vi "The ChapR.vi"(9 "Position":u8=49, 10 "Alliance":u8=66, 11 "TeamNo":u16=2468) -> ()   [LabVIEW 2013]
uses:
  ChapR Packet.ctl
  <vilib>/Instr/_visa.llb/VISA Configure Serial Port (Instr).vi
panel:
  out "error out 3":errorcluster
  in  "connection ID":refnum<k16>
  out "error out 2":errorcluster
  out "# elements 2":u32
  out "# elements":u32
  out "error out":errorcluster
  out "value 2":T1
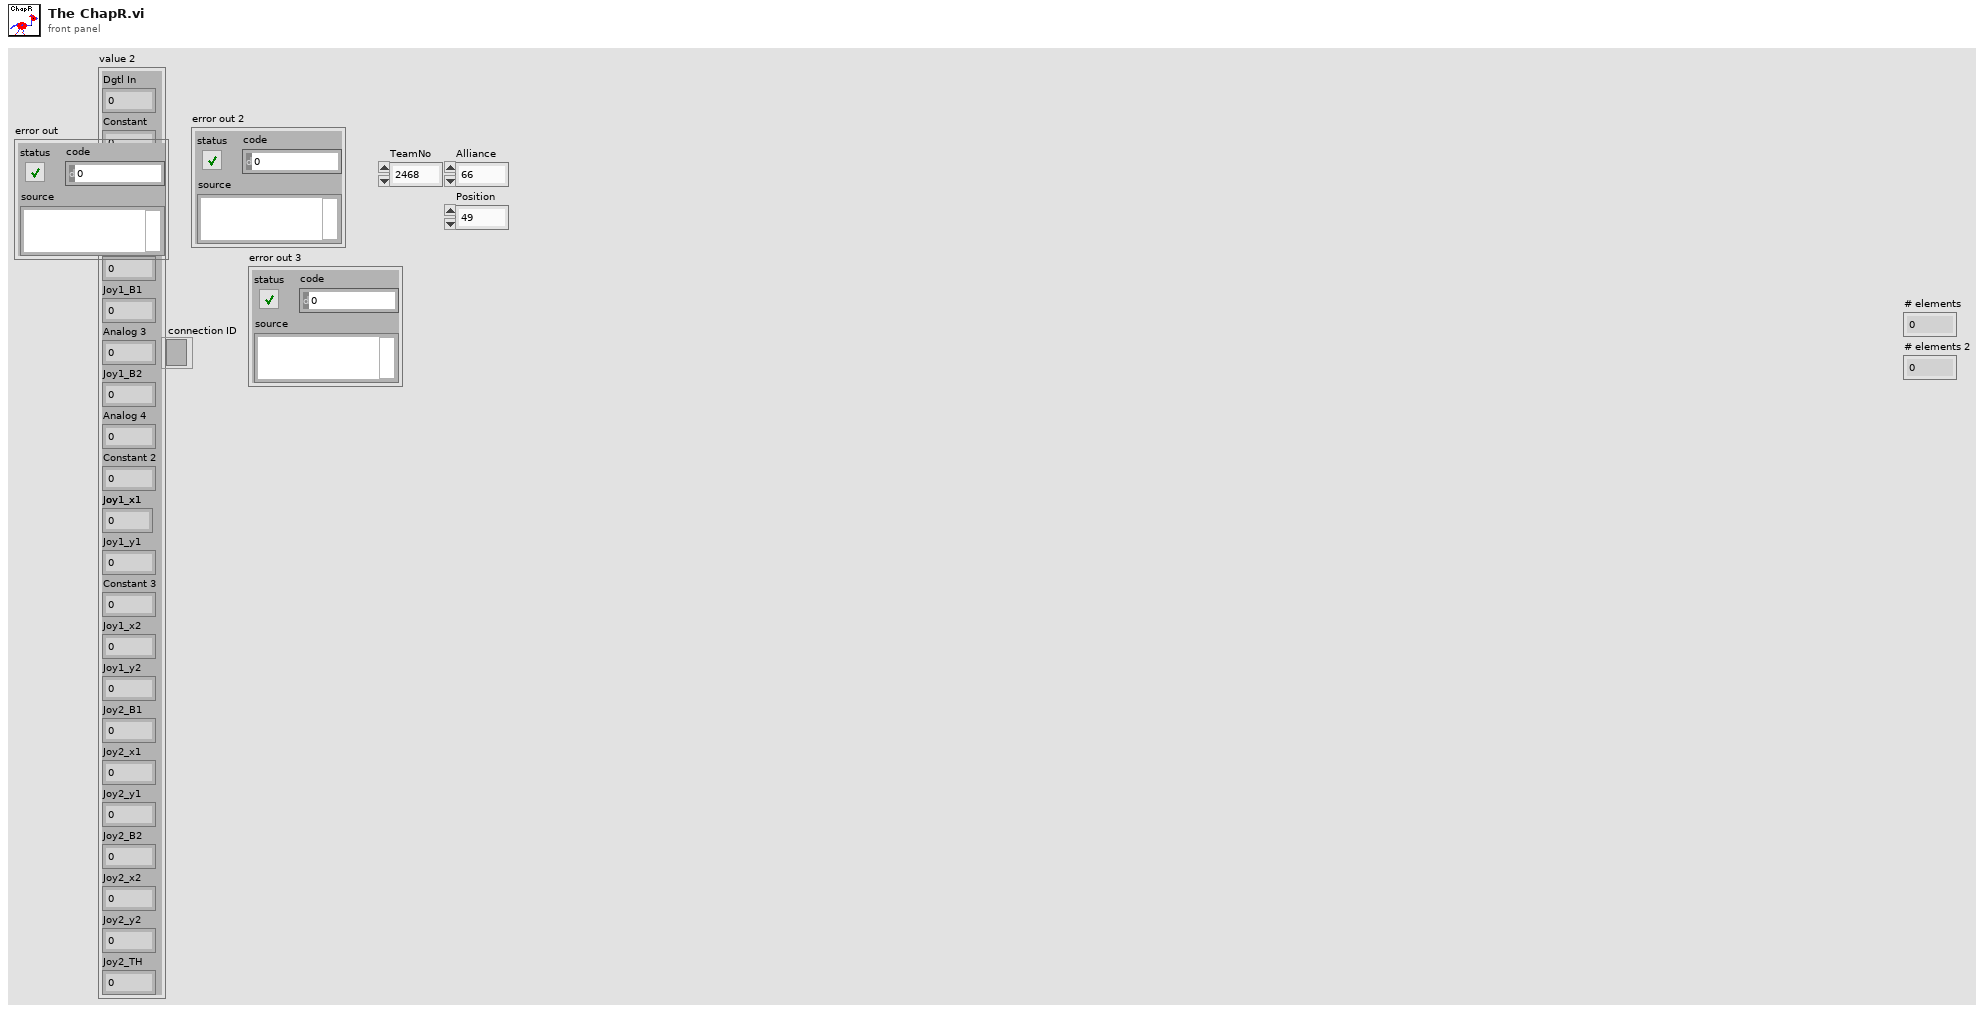
[diagram p1: front panel]
types:
  T1 = typedef "ChapR Packet.ctl" = cluster{"Dgtl In":u8, "Constant":u8, "Analog 1":u16, "Joy1_TH":u8, "Analog 2":u16, "Joy1_B1":u8, "Analog 3":u16, "Joy1_B2":u8, "Analog 4":u16, "Constant 2":u8, "Joy1_x1":i8, "Joy1_y1":i8, "Constant 3":u8, "Joy1_x2":i8, "Joy1_y2":i8, "Joy2_B1":u8, "Joy2_x1":i8, "Joy2_y1":i8, "Joy2_B2":u8, "Joy2_x2":i8, "Joy2_y2":i8, "Joy2_TH":u8}
  T2 = cluster{"read mode":enum16{"polling", "blocking"}, "write mode":enum16{"polling", "blocking"}}
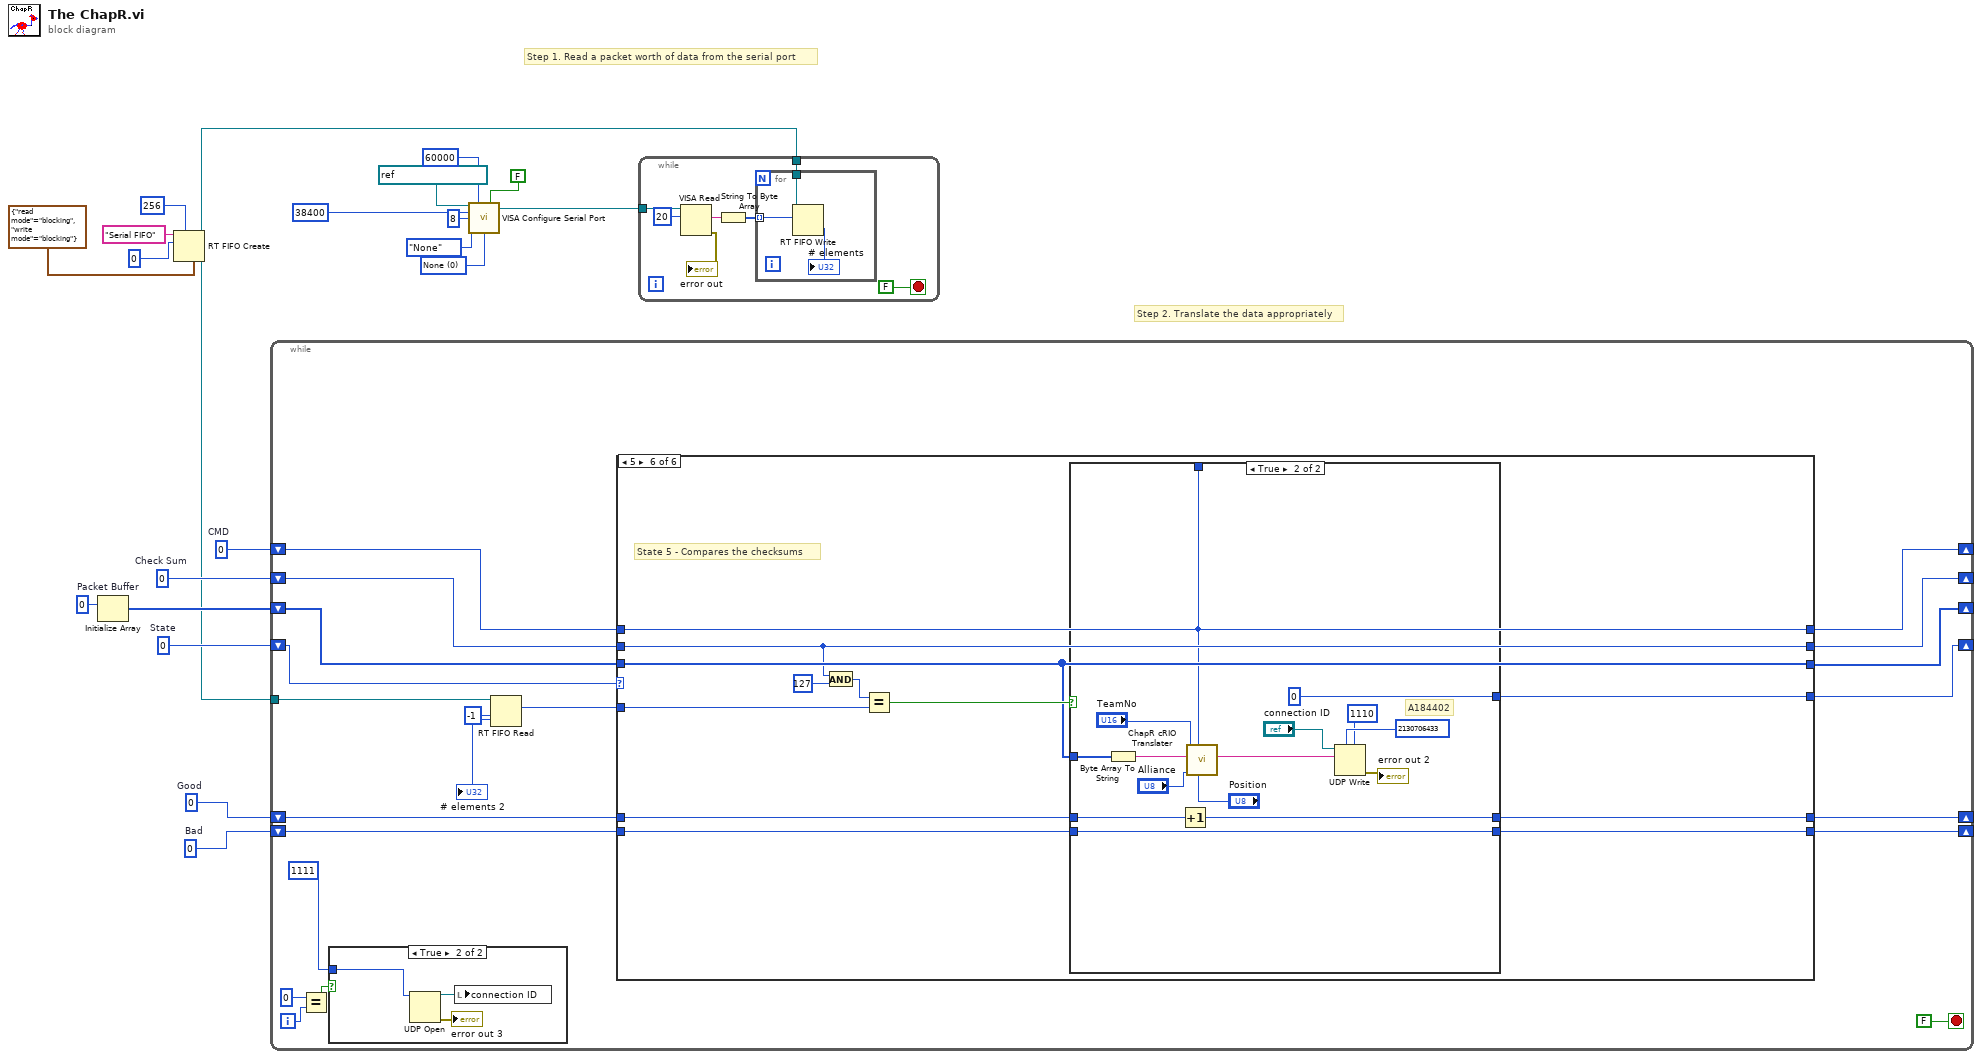
[diagram p0: block diagram]
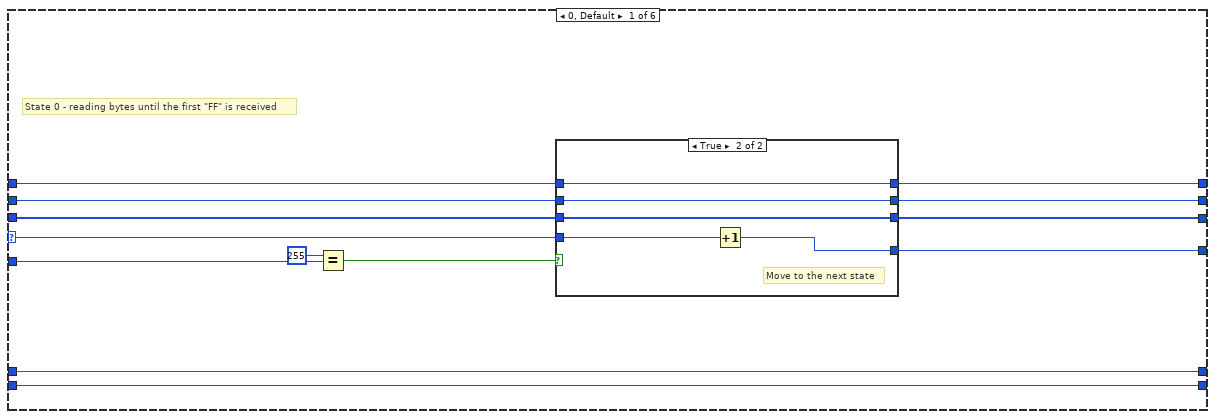
[diagram p3: hidden frame]
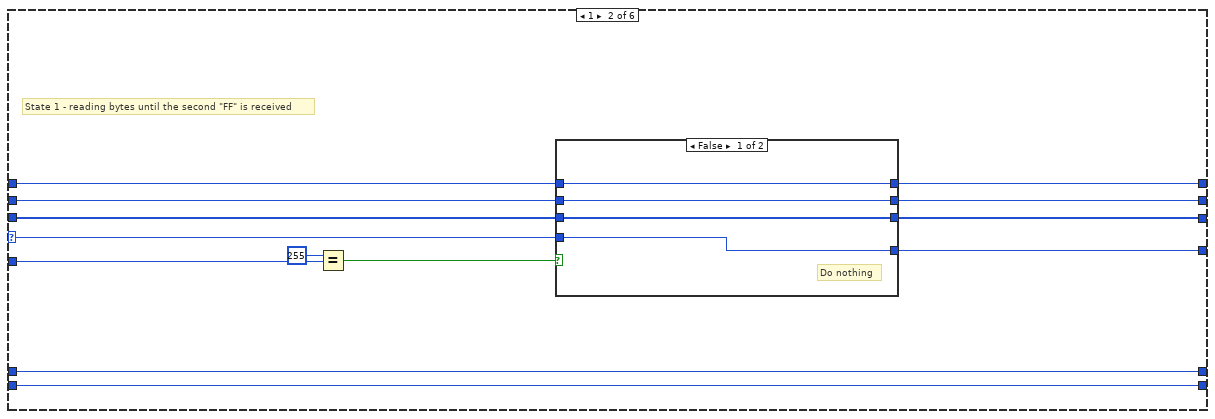
[diagram p5: hidden frame]
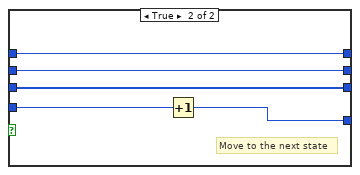
[diagram p6: hidden frame]
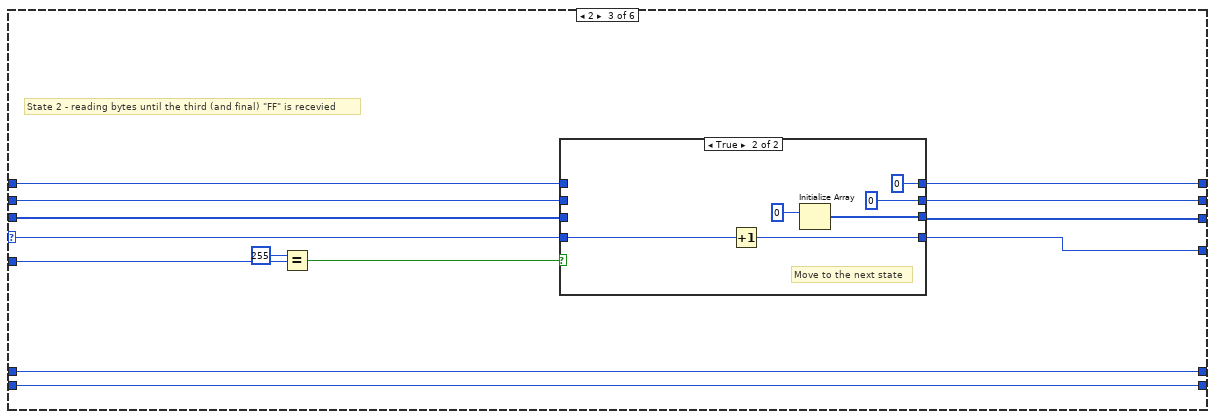
[diagram p7: hidden frame]
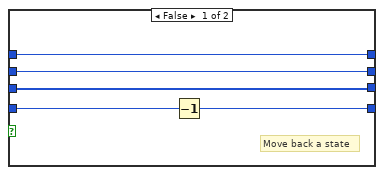
[diagram p8: hidden frame]
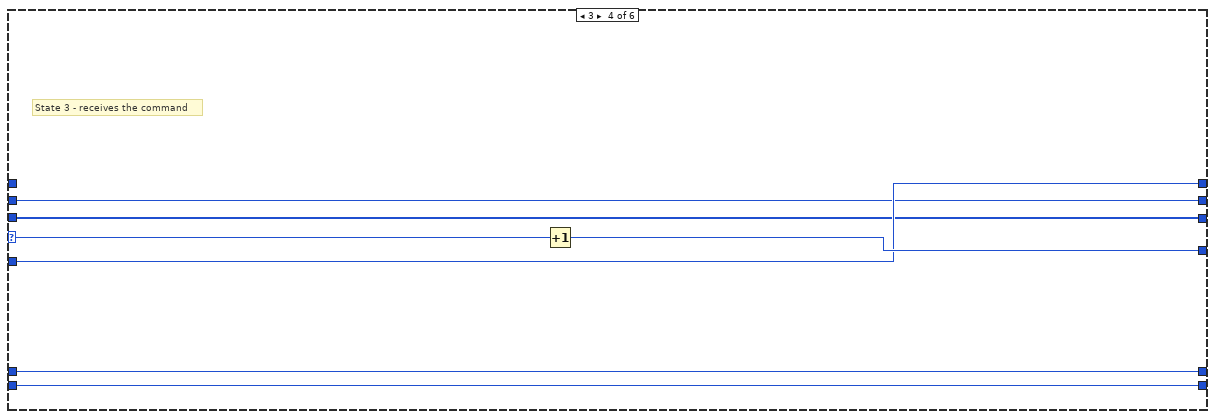
[diagram p9: hidden frame]
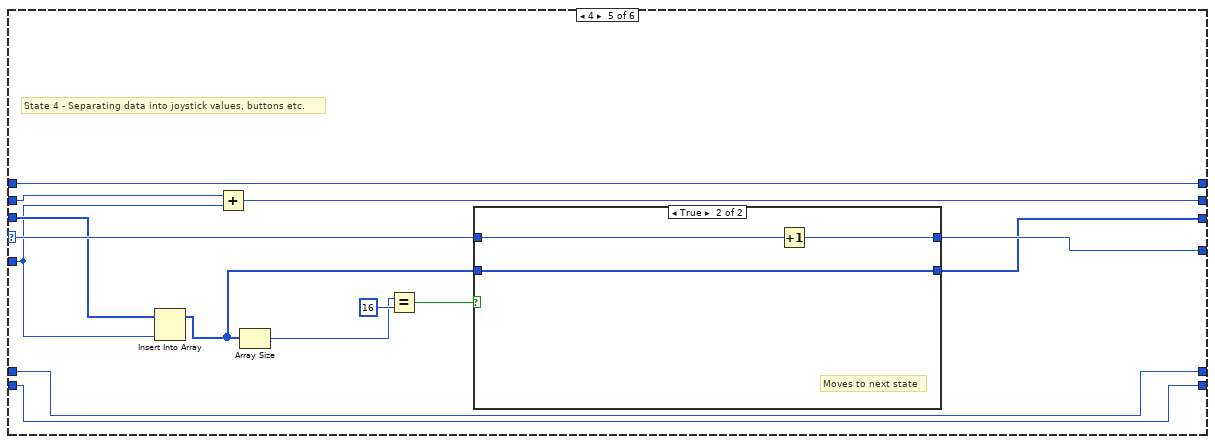
[diagram p10: hidden frame]
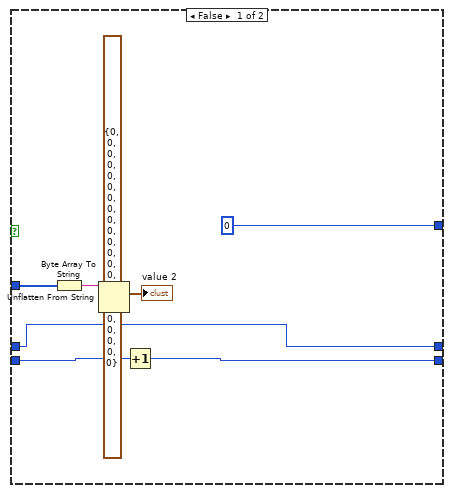
[diagram p12: hidden frame]
diagram:
  w5 = 0  # Bad
  w6 = 0  # Good
  w19 = u16 0 items=["None", "XON/XOFF", "RTS/CTS", "XON/XOFF & RTS/CTS", "DTR/DSR", "XON/XOFF & DTR/DSR"] ("flow control (0:none)")
  w3 = u8 0  # CMD
  w4 = u8 0  # Check Sum
  w20 = 0  # State
  # "Step 2. Translate the data appropriately"
  # "Step 1. Read a packet worth of data from the serial port"
  n1 = Initialize Array "Packet Buffer"(u8 0 ("element")) -> (w8:u8[])  [unwired: 1 in]
  n2 = RT FIFO Create(0:"Serial FIFO" ("name (unnamed)"), 1:u8 0 ("datapoints in waveform (1)"), 4:u32 256 ("size (10)"), 7:T2 {"read mode"=enum."blocking", "write mode"=enum."blocking"} ("r/w modes (polling,polling)")) -> (8:w1:refnum<k33>)  [unwired: 4 in, 2 out]
  n3 = while {
    shift-right: [w39] -> _
    shift-left: w20 -> [w40]
    shift-right: [w29] -> _
    shift-left: w4 -> [w30]
    tunnel: w1 -> [w37]
    shift-right: [w35] -> _
    shift-left: w8 -> [w36]
    shift-right: [w31] -> _
    shift-left: w6 -> [w34]
    shift-right: [w32] -> _
    shift-left: w5 -> [w33]
    shift-right: [w27] -> _
    shift-left: w3 -> [w28]
    i -> [w23]
    stop <- FALSE stop-if-true
    n4 = Equal?(x=0, y=w23) -> (x = y?=w24:bool)
    n5 = case shown="True" w24 {
      tunnel: u16 1111 ("port") -> [_ w43]
      frame False {
      }
      frame True {
        n6 = UDP Open(11:w43) -> (port=w44:refnum<k16>, 0:→"error out 3":errorcluster)  [unwired: 4 in, 1 out]
        n7 = local write "connection ID"(w44) -> ()
      }
    }
    n8 = RT FIFO Read(0:w37, 2:-1 ("timeout in ms (0)")) -> (7:→"# elements 2":u32, 9:w38:u8)  [unwired: 2 in, 3 out]
    n9 = case shown="5" w40 {
      selector: w40 -> [w56 w78 w101 w119 w132 _]
      tunnel: [w55 w77 w100 w118 w133 w149] -> w39
      tunnel: [w47 w69 w91 w113 w130 w140] -> w29
      tunnel: [w45 w67 w89 w117 w120 w139] -> w27
      tunnel: w38 -> [w53 w75 w97 w117 w128 w146]
      tunnel: w36 -> [w52 w74 w95 w116 w129 w145]
      tunnel: [w51 w73 w96 w116 w124 w145] -> w35
      tunnel: w34 -> [w50 w72 w94 w115 w123 w142]
      tunnel: w33 -> [w49 w71 w93 w114 w122 w144]
      tunnel: [w49 w71 w93 w114 w122 w143] -> w32
      tunnel: [w50 w72 w94 w115 w123 w141] -> w31
      tunnel: w30 -> [w48 w70 w92 w113 w121 w140]
      tunnel: w28 -> [w46 w68 w90 _ w120 w139]
      frame 0, Default {
        # "State 0 - reading bytes until the first \"FF\" is received"
        n10 = Equal?(x=u8 255, y=w53) -> (x = y?=w57:bool)
        n11 = case shown="True" w57 {
          tunnel: w56 -> [w61 w66]
          tunnel: [w61 w65] -> w55
          tunnel: w52 -> [w60 w64]
          tunnel: [w60 w64] -> w51
          tunnel: [w59 w63] -> w47
          tunnel: w48 -> [w59 w63]
          tunnel: [w58 w62] -> w45
          tunnel: w46 -> [w58 w62]
          frame False {
            # "Do nothing"
          }
          frame True {
            # "Move to the next state"
            n12 = Increment(x=w66) -> (x+1=w65:i32)
          }
        }
      }
      frame 1 {
        # "State 1 - reading bytes until the second \"FF\" is received"
        n13 = Equal?(x=u8 255, y=w75) -> (x = y?=w79:bool)
        n14 = case shown="False" w79 {
          tunnel: w78 -> [w83 w88]
          tunnel: [w83 w87] -> w77
          tunnel: w74 -> [w82 w86]
          tunnel: [w82 w86] -> w73
          tunnel: [w81 w85] -> w69
          tunnel: w70 -> [w81 w85]
          tunnel: [w80 w84] -> w67
          tunnel: w68 -> [w80 w84]
          frame False {
            # "Do nothing"
          }
          frame True {
            # "Move to the next state"
            n15 = Increment(x=w88) -> (x+1=w87:i32)
          }
        }
      }
      frame 2 {
        # "State 2 - reading bytes until the third (and final) \"FF\" is recevied"
        n16 = Equal?(x=u8 255, y=w97) -> (x = y?=w98:bool)
        n17 = case shown="True" w98 {
          tunnel: [w105 w111] -> w100
          tunnel: w101 -> [w106 w112]
          tunnel: [w103 u8 0] -> w91
          tunnel: [w102 u8 0] -> w89
          tunnel: [w104 w107] -> w96
          tunnel: w95 -> [w104 _]
          tunnel: w92 -> [w103 _]
          tunnel: w90 -> [w102 _]
          frame False {
            # "Move back a state"
            n18 = Decrement(x=w106) -> (x-1=w105:i32)
          }
          frame True {
            # "Move to the next state"
            n19 = Increment(x=w112) -> (x+1=w111:i32)
            n20 = Initialize Array ("Packet Buffer")(u8 0 ("element")) -> (w107:u8[])  [unwired: 1 in]
          }
        }
      }
      frame 3 {
        # "State 3 - receives the command"
        n21 = Increment(x=w119) -> (x+1=w118:i32)
      }
      frame 4 {
        # "State 4 - Separating data into joystick values, buttons etc."
        n22 = Insert Into Array(array=w129, new element=w128) -> (w125:u8[])  [unwired: 1 in]
        n23 = Add(x=w121, y=w128) -> (x+y=w130:u8)
        n24 = Array Size(array=w125) -> (size(s)=w127:i32)
        n25 = Equal?(x=w127, y=16) -> (x = y?=w126:bool)
        n26 = case shown="True" w126 {
          tunnel: [w135 w137] -> w133
          tunnel: w132 -> [w135 w138]
          tunnel: w125 -> [w134 w136]
          tunnel: [w134 w136] -> w124
          frame False {
            # "Do nothing"
          }
          frame True {
            # "Moves to next state"
            n27 = Increment(x=w138) -> (x+1=w137:i32)
          }
        }
      }
      frame 5 {
        # "State 5 - Compares the checksums"
        n28 = And(x=w140, y=u8 127) -> (x .and. y?=w148:u8)
        n29 = Equal?(x=w148, y=w146) -> (x = y?=w150:bool)
        n30 = case shown="True" w150 {
          tunnel: [0 0] -> w149
          tunnel: w145 -> [w156 w172]
          tunnel: w144 -> [w154 w171]
          tunnel: [w153 w171] -> w143
          tunnel: w142 -> [w152 w170]
          tunnel: [w152 w169] -> w141
          tunnel: w139 -> [_ w159]
          frame False {
            n31 = Byte Array To String(unsigned byte array=w156) -> (string=w155:string)
            n32 = Unflatten From String(type=T1 {"Dgtl In"=0, "Constant"=0, "Analog 1"=0, "Joy1_TH"=0, "Analog 2"=0, "Joy1_B1"=0, "Analog 3"=0, "Joy1_B2"=0, "Analog 4"=0, "Constant 2"=0, "Joy1_x1"=0, "Joy1_y1"=0, "Constant 3"=0, "Joy1_x2"=0, "Joy1_y2"=0, "Joy2_B1"=0, "Joy2_x1"=0, "Joy2_y1"=0, "Joy2_B2"=0, "Joy2_x2"=0, "Joy2_y2"=0, "Joy2_TH"=0}, binary string=w155) -> (value=→"value 2":T1)  [unwired: 3 in, 2 out]
            n33 = Increment(x=w154) -> (x+1=w153:i32)
          }
          frame True {
            # "A184402"
            n34 = Byte Array To String(unsigned byte array=w172) -> (string=w168:string)
            n35 = Increment(x=w170) -> (x+1=w169:i32)
            n36 = call "ChapR cRIO Translater.vi"("Position"="Position", "CMD"=w159, "Alliance"="Alliance", "ChapR Data"=w168, "TeamNo"="TeamNo") -> ("Network Data"=w162:string)  [unwired: 6 in]
            n37 = UDP Write(address=u32 2130706433 ("net address"), port or service name=u16 1110, connection ID="connection ID", data in=w162) -> (error out=→"error out 2":errorcluster)  [unwired: 2 in, 1 out]
          }
        }
      }
    }
  }
  n38 = call-poly "VISA Configure Serial Port"("VISA resource name"=refnum<visa-resource-name> "ASRL1::INSTR", "timeout (10sec)"=u32 60000, "Enable Termination\nChar (T)"=FALSE ("Enable Termination\nChar (T)"), "baud rate (9600)"=u32 38400, "data bits (8)"=u16 8, "parity (0:none)"=enum16{"None", "Odd", "Even", "Mark", "Space"}."None", "flow control (0:none)"=w19) -> ("VISA resource name out"=w12:refnum<visa-resource-name>)  [unwired: 7 in, 1 out]
  n39 = while {
    tunnel: w12 -> [w179]
    tunnel: w1 -> [w177]
    stop <- FALSE stop-if-true
    n40 = VISA Read(VISA resource name=w179, byte count=u32 20) -> (read buffer=w175:string, error out=→"error out":errorcluster)  [unwired: 1 in, 2 out]
    n41 = String To Byte Array(string=w175) -> (unsigned byte array=w176:u8[])
    n42 = for {
      tunnel: w177 -> [w183]
      tunnel: w176 -> [w182] mode=indexing
      n43 = RT FIFO Write(0:w183, 1:w182) -> (7:→"# elements":u32)  [unwired: 3 in, 3 out]
    }
  }
